vi "moveKnot.vi"(9 "knot":cluster{"X":i32, "Y":i32}, 11 "head":cluster{"X":i32, "Y":i32}) -> (1 "knot":cluster{"X":i32, "Y":i32})   [LabVIEW 2023]
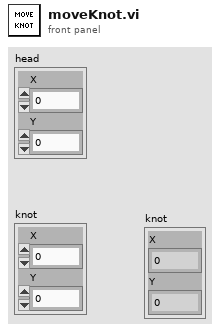
[diagram p1: front panel]
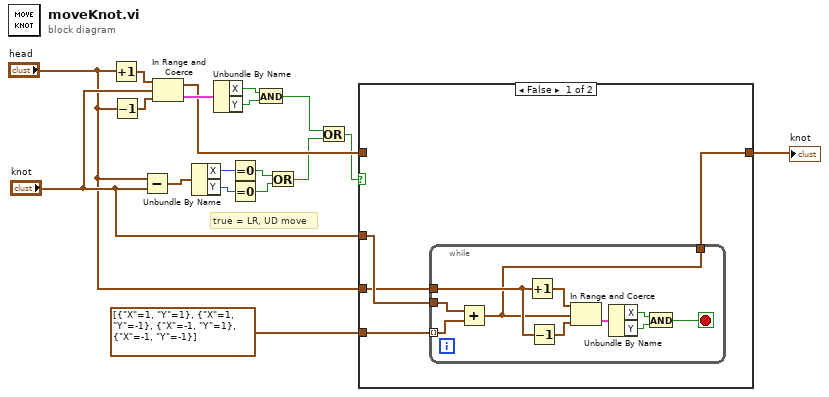
[diagram p0: block diagram]
diagram:
  # "true = LR, UD move"
  n1 = Increment(x="head") -> (x+1=w18:cluster{"X":i32, "Y":i32})
  n2 = Decrement(x="head") -> (x-1=w17:cluster{"X":i32, "Y":i32})
  n3 = Subtract(x="head", y="knot") -> (x-y=w15:cluster{"X":i32, "Y":i32})
  n4 = In Range and Coerce(upper limit=w18, x="knot", lower limit=w17) -> (coerced(x)=w10:cluster{"X":i32, "Y":i32}, In Range?=w16:cluster{"X":bool, "Y":bool})
  n5 = Unbundle By Name(w15) -> ("X"=w14:i32, "Y"=w13:i32)
  n6 = Unbundle By Name(w16) -> ("X"=w4:bool, "Y"=w5:bool)
  n7 = Equal To 0?(x=w14) -> (x = 0?=w12:bool)
  n8 = Equal To 0?(x=w13) -> (x = 0?=w11:bool)
  n9 = And(x=w4, y=w5) -> (x .and. y?=w3:bool)
  n10 = Or(x=w12, y=w11) -> (x .or. y?=w2:bool)
  n11 = Or(x=w3, y=w2) -> (x .or. y?=w1:bool)
  n12 = case shown="False" w1 {
    tunnel: [w19 w33] -> w6
    tunnel: w10 -> [_ w33]
    tunnel: "knot" -> [w21 _]
    tunnel: cluster{"X":i32, "Y":i32}[] [{"X"=1, "Y"=1}, {"X"=1, "Y"=-1}, {"X"=-1, "Y"=1}, {"X"=-1, "Y"=-1}] ("initialized array") -> [w22 _]
    tunnel: "head" -> [w20 _]
    frame False {
      n13 = while {
        tunnel: w22 -> [w31] mode=indexing
        tunnel: w21 -> [w32]
        tunnel: w20 -> [w29]
        tunnel: [w23] -> w19
        stop <- w24 stop-if-true
        n14 = Add(x=w32, y=w31) -> (x+y=w23:cluster{"X":i32, "Y":i32})
        n15 = Increment(x=w29) -> (x+1=w30:cluster{"X":i32, "Y":i32})
        n16 = Decrement(x=w29) -> (x-1=w28:cluster{"X":i32, "Y":i32})
        n17 = In Range and Coerce(upper limit=w30, x=w23, lower limit=w28) -> (In Range?=w27:cluster{"X":bool, "Y":bool})  [unwired: 1 out]
        n18 = Unbundle By Name(w27) -> ("X"=w26:bool, "Y"=w25:bool)
        n19 = And(x=w26, y=w25) -> (x .and. y?=w24:bool)
      }
    }
    frame True {
    }
  }
  "knot" <- w6
